vi "AsciiStringToHexString.vi"(1 "输入Asciistring1":string) -> (0 "输出HexString":string)   [LabVIEW 2020]
panel:
  out "输出数组1":u8[](array[numeric])
  out "输出数组":u8[](array[numeric])
  out "low":u8
  out "high":u8
  in  "输入Asciistring":string
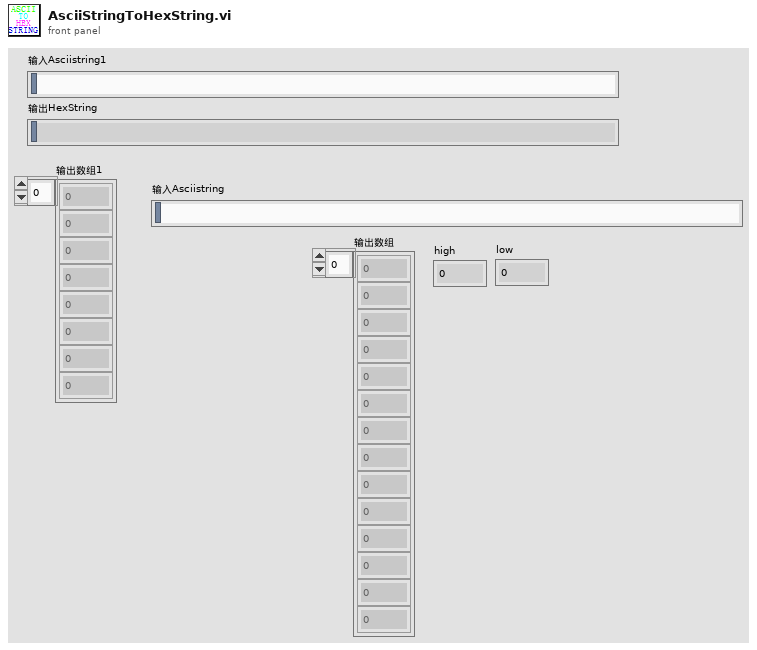
[diagram p1: front panel]
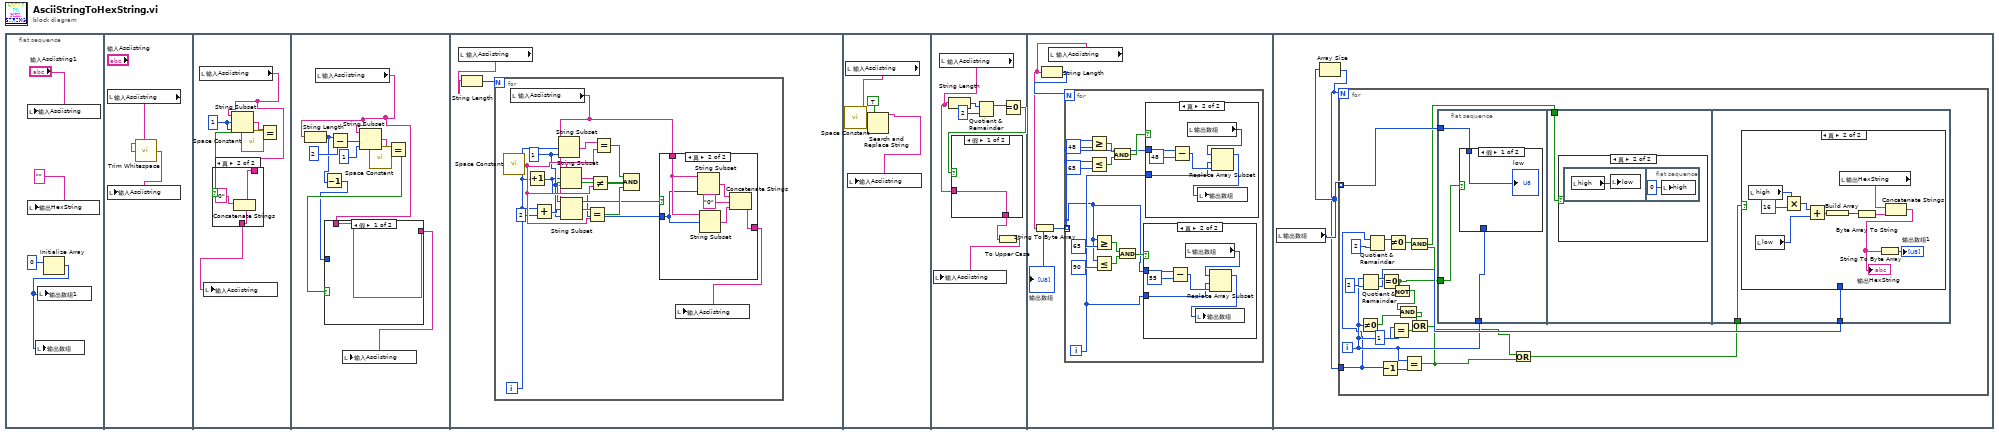
[diagram p0: block diagram]
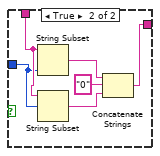
[diagram p3: hidden frame]
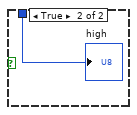
[diagram p8: hidden frame]
diagram:
  n1 = flat-sequence {
    frame #0 {
      n2 = local write "输入Asciistring"("输入Asciistring1") -> ()
      n3 = local write "输出HexString"("" ("输出HexString")) -> ()
      n4 = Initialize Array(u8 0 ("元素")) -> (w2:u8[])  [unwired: 1 in]
      n5 = local write "输出数组"(w2) -> ()
      n6 = local write "输出数组1"(w2) -> ()
    }
    frame #1 {
      n7 = local read "输入Asciistring"() -> (w6:string)
      n8 = call <vilib>:"Trim Whitespace.vi"("string"=w6) -> ("trimmed string"=w5:string)  [unwired: 1 in]
      n9 = local write "输入Asciistring"(w5) -> ()
    }
    frame #2 {
      w12 = 1 ("偏移量(0)")
      n10 = local read "输入Asciistring"() -> (w8:string)
      n11 = String Subset(string=w8, offset (0)=w12, length (rest)=w12) -> (substring=w11:string)
      n12 = call <vilib>:"Space Constant.vi"() -> ("String"=w10:string)
      n13 = Equal?(x=w11, y=w10) -> (x = y?=w9:bool)
      n14 = case shown="真" w9 {
        tunnel: w8 -> [w13 w15]
        tunnel: [w13 w14] -> w7
        frame False {
        }
        frame True {
          n15 = Concatenate Strings("0" ("字符串"), w15) -> (w14:string)
        }
      }
      n16 = local write "输入Asciistring"(w7) -> ()
    }
    frame #3 {
      n17 = local read "输入Asciistring"() -> (w18:string)
      n18 = String Length(string=w18) -> (length=w20:i32)
      n19 = Decrement(x=w20) -> (x-1=w19:i32)
      n20 = Subtract(x=w20, y=2) -> (x-y=w22:i32)
      n21 = String Subset(string=w18, offset (0)=w22, length (rest)=1 ("y")) -> (substring=w24:string)
      n22 = call <vilib>:"Space Constant.vi"() -> ("String"=w25:string)
      n23 = Equal?(x=w24, y=w25) -> (x = y?=w26:bool)
      n24 = case shown="假" w26 {
        tunnel: w18 -> [w27 w32]
        tunnel: [w27 w33] -> w17
        tunnel: w19 -> [_ w31]
        frame False {
        }
        frame True {
          n25 = String Subset(string=w32, length (rest)=w31) -> (substring=w30:string)  [unwired: 1 in]
          n26 = String Subset(string=w32, offset (0)=w31) -> (substring=w28:string)  [unwired: 1 in]
          n27 = Concatenate Strings(w30, "0" ("字符串"), w28) -> (w33:string)
        }
      }
      n28 = local write "输入Asciistring"(w17) -> ()
    }
    frame #4 {
      n29 = local read "输入Asciistring"() -> (w34:string)
      n30 = String Length(string=w34) -> (length=w35:i32)
      n31 = for {
        N: w35 -> [_]
        i -> [w41]
        w39 = 1 ("长度（剩余）")
        n32 = call <vilib>:"Space Constant.vi"() -> ("String"=w47:string)
        n33 = local read "输入Asciistring"() -> (w36:string)
        n34 = Increment(x=w41) -> (x+1=w38:i32)
        n35 = Add(x=w41, y=2) -> (x+y=w42:i32)
        n36 = String Subset(string=w36, offset (0)=w41, length (rest)=w39) -> (substring=w50:string)
        n37 = String Subset(string=w36, offset (0)=w38, length (rest)=w39) -> (substring=w48:string)
        n38 = String Subset(string=w36, offset (0)=w42, length (rest)=w39) -> (substring=w49:string)
        n39 = Equal?(x=w49, y=w47) -> (x = y?=w44:bool)
        n40 = Not Equal?(x=w48, y=w47) -> (x != y?=w45:bool)
        n41 = Equal?(x=w50, y=w47) -> (x = y?=w46:bool)
        n42 = Compound Arithmetic op=AND(w46, w45, w44) -> (w43:bool)
        n43 = case shown="真" w43 {
          tunnel: w38 -> [_ w56]
          tunnel: w36 -> [w51 w57]
          tunnel: [w51 w52] -> w37
          frame False {
          }
          frame True {
            n44 = String Subset(string=w57, length (rest)=w56) -> (substring=w55:string)  [unwired: 1 in]
            n45 = String Subset(string=w57, offset (0)=w56) -> (substring=w53:string)  [unwired: 1 in]
            n46 = Concatenate Strings(w55, "0" ("字符串"), w53) -> (w52:string)
          }
        }
        n47 = local write "输入Asciistring"(w37) -> ()
      }
    }
    frame #5 {
      n48 = call <vilib>:"Space Constant.vi"() -> ("String"=w61:string)
      n49 = local read "输入Asciistring"() -> (w59:string)
      n50 = Search and Replace String(replace all?=TRUE ("替换全部？(F)"), input string=w59, search string=w61) -> (result string=w58:string)  [unwired: 5 in, 3 out]
      n51 = local write "输入Asciistring"(w58) -> ()
    }
    frame #6 {
      n52 = local read "输入Asciistring"() -> (w63:string)
      n53 = String Length(string=w63) -> (length=w68:i32)
      n54 = Quotient & Remainder(x=w68, y=2) -> (x-y*floor(x/y)=w66:i32)  [unwired: 1 out]
      n55 = Equal To 0?(x=w66) -> (x = 0?=w65:bool)
      n56 = case shown="假" w65 {
        tunnel: w63 -> [w69 w70]
        tunnel: [w69 w70] -> w64
        frame False {
        }
        frame True {
        }
      }
      n57 = To Upper Case(1:w64) -> (0:w62:string)
      n58 = local write "输入Asciistring"(w62) -> ()
    }
    frame #7 {
      n59 = local read "输入Asciistring"() -> (w71:string)
      n60 = String To Byte Array(string=w71) -> (unsigned byte array=w72:u8[])
      "输出数组" <- w72
      n61 = String Length(string=w71) -> (length=w73:i32)
      n62 = for {
        N: w73 -> [_]
        tunnel: w72 -> [w74] mode=indexing
        i -> [w75]
        n63 = Greater Or Equal?(x=w74, y=u8 48) -> (x >= y?=w82:bool)
        n64 = Less Or Equal?(x=w74, y=u8 65) -> (x <= y?=w83:bool)
        n65 = Greater Or Equal?(x=w74, y=u8 65) -> (x >= y?=w80:bool)
        n66 = Less Or Equal?(x=w74, y=u8 90) -> (x <= y?=w79:bool)
        n67 = And(x=w82, y=w83) -> (x .and. y?=w81:bool)
        n68 = And(x=w80, y=w79) -> (x .and. y?=w76:bool)
        n69 = case shown="真" w76 {
          tunnel: w74 -> [_ w91]
          tunnel: w75 -> [_ w88]
          frame False {
          }
          frame True {
            n70 = Subtract(x=w91, y=u8 55) -> (x-y=w89:u8)
            n71 = local read "输出数组"() -> (w87:u8[])
            n72 = Replace Array Subset(array=w87, new element=w89, index=w88) -> (w86:u8[])
            n73 = local write "输出数组"(w86) -> ()
          }
        }
        n74 = case shown="真" w81 {
          tunnel: w74 -> [_ w97]
          tunnel: w75 -> [_ w94]
          frame False {
          }
          frame True {
            n75 = Subtract(x=w97, y=u8 48) -> (x-y=w95:u8)
            n76 = local read "输出数组"() -> (w93:u8[])
            n77 = Replace Array Subset(array=w93, new element=w95, index=w94) -> (w92:u8[])
            n78 = local write "输出数组"(w92) -> ()
          }
        }
      }
    }
    frame #8 {
      n79 = local read "输出数组"() -> (w99:u8[])
      n80 = Array Size(array=w99) -> (size(s)=w98:i32)
      n81 = for {
        N: w98 -> [_]
        tunnel: w99 -> [w117] mode=indexing
        tunnel: w98 -> [w103]
        i -> [w109]
        n82 = Not Equal To 0?(x=w109) -> (x != 0?=w116:bool)
        n83 = Quotient & Remainder(x=w109, y=2) -> (x-y*floor(x/y)=w118:i32, floor(x/y)=w115:i32)
        n84 = Quotient & Remainder(x=w103, y=2) -> (x-y*floor(x/y)=w105:i32)  [unwired: 1 out]
        n85 = Decrement(x=w103) -> (x-1=w106:i32)
        n86 = Equal To 0?(x=w118) -> (x = 0?=w110:bool)
        n87 = Not Equal To 0?(x=w105) -> (x != 0?=w102:bool)
        n88 = Equal?(x=w109, y=1) -> (x = y?=w113:bool)
        n89 = Not(x=w110) -> (.not. x?=w111:bool)
        n90 = And(x=w111, y=w116) -> (x .and. y?=w112:bool)
        n91 = Equal?(x=w109, y=w106) -> (x = y?=w101:bool)
        n92 = And(x=w102, y=w101) -> (x .and. y?=w100:bool)
        n93 = Or(x=w112, y=w113) -> (x .or. y?=w108:bool)
        n94 = flat-sequence {
          tunnel: w117 -> [w122]
          tunnel: w109 -> [w121]
          tunnel: w110 -> [w120]
          tunnel: w100 -> [w125]
          tunnel: w115 -> [w129]
          tunnel: w107 -> [w128]
          frame #0 {
            n95 = case shown="假" w120 {
              tunnel: w122 -> [w123 w124]
              tunnel: w121 -> [_ _]
              frame False {
                "low" <- w123
              }
              frame True {
                "high" <- w124
              }
            }
          }
          frame #1 {
            n96 = case shown="真" w125 {
              frame False {
              }
              frame True {
                n97 = flat-sequence {
                  frame #0 {
                    n98 = local read "high"() -> (w126:u8)
                    n99 = local write "low"(w126) -> ()
                  }
                  frame #1 {
                    n100 = local write "high"(u8 0 ("low")) -> ()
                  }
                }
              }
            }
          }
          frame #2 {
            n101 = case shown="真" w128 {
              tunnel: w129 -> [_ _]
              frame False {
              }
              frame True {
                n102 = local read "high"() -> (w139:u8)
                n103 = local read "low"() -> (w136:u8)
                n104 = Multiply(x=w139, y=u8 16) -> (x*y=w137:u8)
                n105 = Add(x=w137, y=w136) -> (x+y=w133:u8)
                n106 = Build Array(w133) -> (w132:u8[])
                n107 = local read "输出HexString"() -> (w134:string)
                n108 = Byte Array To String(unsigned byte array=w132) -> (string=w135:string)
                n109 = Concatenate Strings(w134, w135) -> (w130:string)
                "输出HexString" <- w130
                n110 = String To Byte Array(string=w130) -> (unsigned byte array=→"输出数组1":u8[])
              }
            }
          }
        }
        n111 = Or(x=w108, y=w101) -> (x .or. y?=w107:bool)
      }
    }
  }
